vi "VI Tree.vi"   [LabVIEW 2018, in "LeCroy Wave Series.lvlib"]
doc: "This is the instrument driver for the LeCroy Wave Series Oscilloscopes. The VI Tree displays all the user-callable VIs of the instrument driver in an organized table."
uses:
  LeCroy Wave Series.lvlib
  Data/Read Single Waveform.vi
  Configure/Configure Edge Trigger.vi
  Data/Read Waveform Measurement (Standard).vi
panel:
  # "(c) 2008 - 2012 NATIONAL INSTRUMENTS.  ALL RIGHTS RESERVED."
  # "SEE DIAGRAM\nFOR VI TREE."
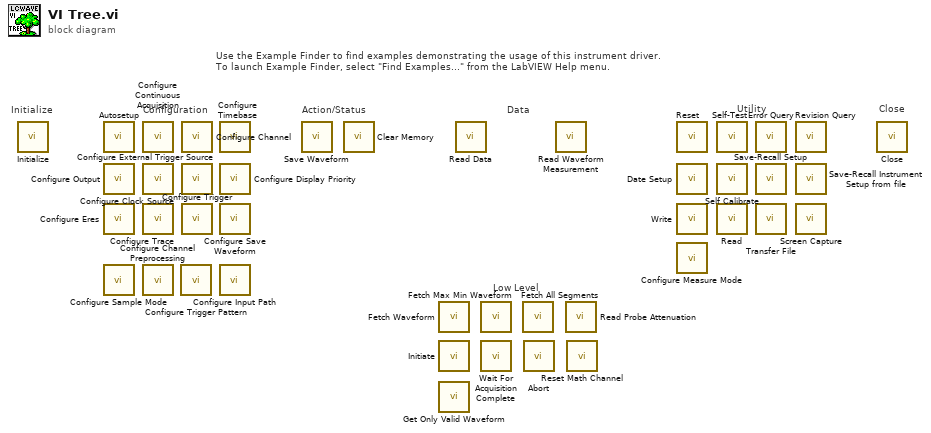
[diagram p0: block diagram]
diagram:
  # "Low Level"
  # "Action/Status"
  # "Use the Example Finder to find examples demonstrating the usage of this instrument driver.\nTo launch Example Finder, select \"Find Examples...\" from the LabVIEW Help menu."
  # "Configuration"
  # "Utility"
  # "Data"
  # "Close"
  # "Initialize"
  n1 = call "Initialize.vi"() -> ()  [unwired: 10 in, 2 out]
  n2 = call "Autosetup.vi"() -> ()  [unwired: 10 in, 2 out]
  n3 = call "Configure Output.vi"() -> ()  [unwired: 14 in, 2 out]
  n4 = call "Configure Eres.vi"() -> ()  [unwired: 10 in, 2 out]
  n5 = call "Configure Sample Mode.vi"() -> ()  [unwired: 10 in, 2 out]
  n6 = call "Configure Continuous Acquisition.vi"() -> ()  [unwired: 10 in, 2 out]
  n7 = call "Configure Clock Source.vi"() -> ()  [unwired: 10 in, 2 out]
  n8 = call "Configure Trace.vi"() -> ()  [unwired: 10 in, 2 out]
  n9 = call "Configure Channel Preprocessing.vi"() -> ()  [unwired: 14 in, 2 out]
  n10 = call "Configure Trigger Pattern.vi"() -> ()  [unwired: 18 in, 2 out]
  n11 = call "Configure Channel.vi"() -> ()  [unwired: 14 in, 2 out]
  n12 = call "Configure External Trigger Source.vi"() -> ()  [unwired: 10 in, 2 out]
  n13 = call-poly "Configure Trigger.vi"() -> ()  [unwired: 14 in, 2 out]
  n14 = call "Configure Timebase.vi"() -> ()  [unwired: 10 in, 2 out]
  n15 = call "Configure Display Priority.vi"() -> ()  [unwired: 10 in, 2 out]
  n16 = call "Configure Save Waveform.vi"() -> ()  [unwired: 18 in, 2 out]
  n17 = call "Configure Input Path.vi"() -> ()  [unwired: 14 in, 2 out]
  n18 = call "Save Waveform.vi"() -> ()  [unwired: 9 in, 3 out]
  n19 = call "Clear Memory.vi"() -> ()  [unwired: 10 in, 2 out]
  n20 = call "Fetch Waveform.vi"() -> ()  [unwired: 9 in, 3 out]
  n21 = call "Initiate.vi"() -> ()  [unwired: 10 in, 2 out]
  n22 = call "Get Only Valid Waveform.vi"() -> ()  [unwired: 11 in, 1 out]
  n23 = call-poly "Read Data.vi"() -> ()  [unwired: 9 in, 3 out]
  n24 = call "Fetch Max Min Waveform.vi"() -> ()  [unwired: 8 in, 4 out]
  n25 = call "Wait For Acquisition Complete.vi"() -> ()  [unwired: 9 in, 3 out]
  n26 = call "Fetch All Segments.vi"() -> ()  [unwired: 9 in, 3 out]
  n27 = call "Abort.vi"() -> ()  [unwired: 10 in, 2 out]
  n28 = call-poly "Read Waveform Measurement.vi"() -> ()  [unwired: 12 in, 4 out]
  n29 = call "Read Probe Attenuation.vi"() -> ()  [unwired: 9 in, 3 out]
  n30 = call "Reset Math Channel.vi"() -> ()  [unwired: 10 in, 2 out]
  n31 = call "Reset.vi"() -> ()  [unwired: 10 in, 2 out]
  n32 = call "Date Setup.vi"() -> ()  [unwired: 14 in, 2 out]
  n33 = call "Write.vi"() -> ()  [unwired: 10 in, 2 out]
  n34 = call "Configure Measure Mode.vi"() -> ()  [unwired: 14 in, 2 out]
  n35 = call "Self-Test.vi"() -> ()  [unwired: 8 in, 4 out]
  n36 = call "Self Calibrate.vi"() -> ()  [unwired: 10 in, 2 out]
  n37 = call "Read.vi"() -> ()  [unwired: 8 in, 4 out]
  n38 = call "Error Query.vi"() -> ()  [unwired: 8 in, 4 out]
  n39 = call "Save-Recall Setup.vi"() -> ()  [unwired: 10 in, 2 out]
  n40 = call "Transfer File.vi"() -> ()  [unwired: 9 in, 3 out]
  n41 = call "Revision Query.vi"() -> ()  [unwired: 8 in, 4 out]
  n42 = call "Save-Recall Instrument Setup from file.vi"() -> ()  [unwired: 14 in, 2 out]
  n43 = call "Screen Capture.vi"() -> ()  [unwired: 10 in, 2 out]
  n44 = call "Close.vi"() -> ()  [unwired: 11 in, 1 out]
